vi "obwiednia_final.vi"() -> ()   [LabVIEW 2012]
uses:
  <vilib>/Analysis/3filter.llb/FIR Filter (DBL).vi
  <vilib>/Analysis/baseanly.llb/Mean (DBL).vi
  <vilib>/Utility/file.llb/Read From Spreadsheet File (DBL).vi
  <vilib>/addons/Sound and Vibration/Order Analysis/Fault Analysis/SVPO Envelope Detection (1 Ch DBL Array).vi
  <vilib>/Utility/file.llb/Write To Spreadsheet File (DBL).vi
  <vilib>/Analysis/4window.llb/Hamming Window (DBL).vi
  <vilib>/Analysis/NI_AALBase.lvlib
  <vilib>/Analysis/NI_AALPro.lvlib
  <vilib>/Analysis/NI_AAL_SigProc.lvlib
  <vilib>/addons/Sound and Vibration/Order Analysis/Fault Analysis/SoundVib_FaultAnalysis.lvlib
  <vilib>/gmath/NI_Gmath.lvlib
panel:
  out "Rozpoznano":bool
  out "Maks. indeks":i32
  out "Największy wsp.":dbl
  out "Współczynniki":dbl[](array[numeric])
  out "Odległość":dbl[](array[numeric])
  out "Waveform Graph 3":dbl[](graph)
  in  "Liczenie":bool
  in  "Pomiar":bool
  in  "stop":bool
  out "Signal energy":dbl
  out "Frames":dbl[][](array[numeric])
  out "Przekroczenie progu":bool
  out "Tablica ramek":dbl[](graph)
  out "number of columns":i32
  out "number of rows":i32
  out "Threshold Energy":dbl
  out "Diagram energii":dbl[](graph)
  out "size(s)":i32
  out "sum":dbl
  out "Length":dbl
  out "\"Wygładzona\" energia":dbl[](graph)
  out "max index":dbl
  out "min index":dbl
  out "Wypowiedź":dbl[](graph)
  out "Mowa":waveform(dbl)[](graph)
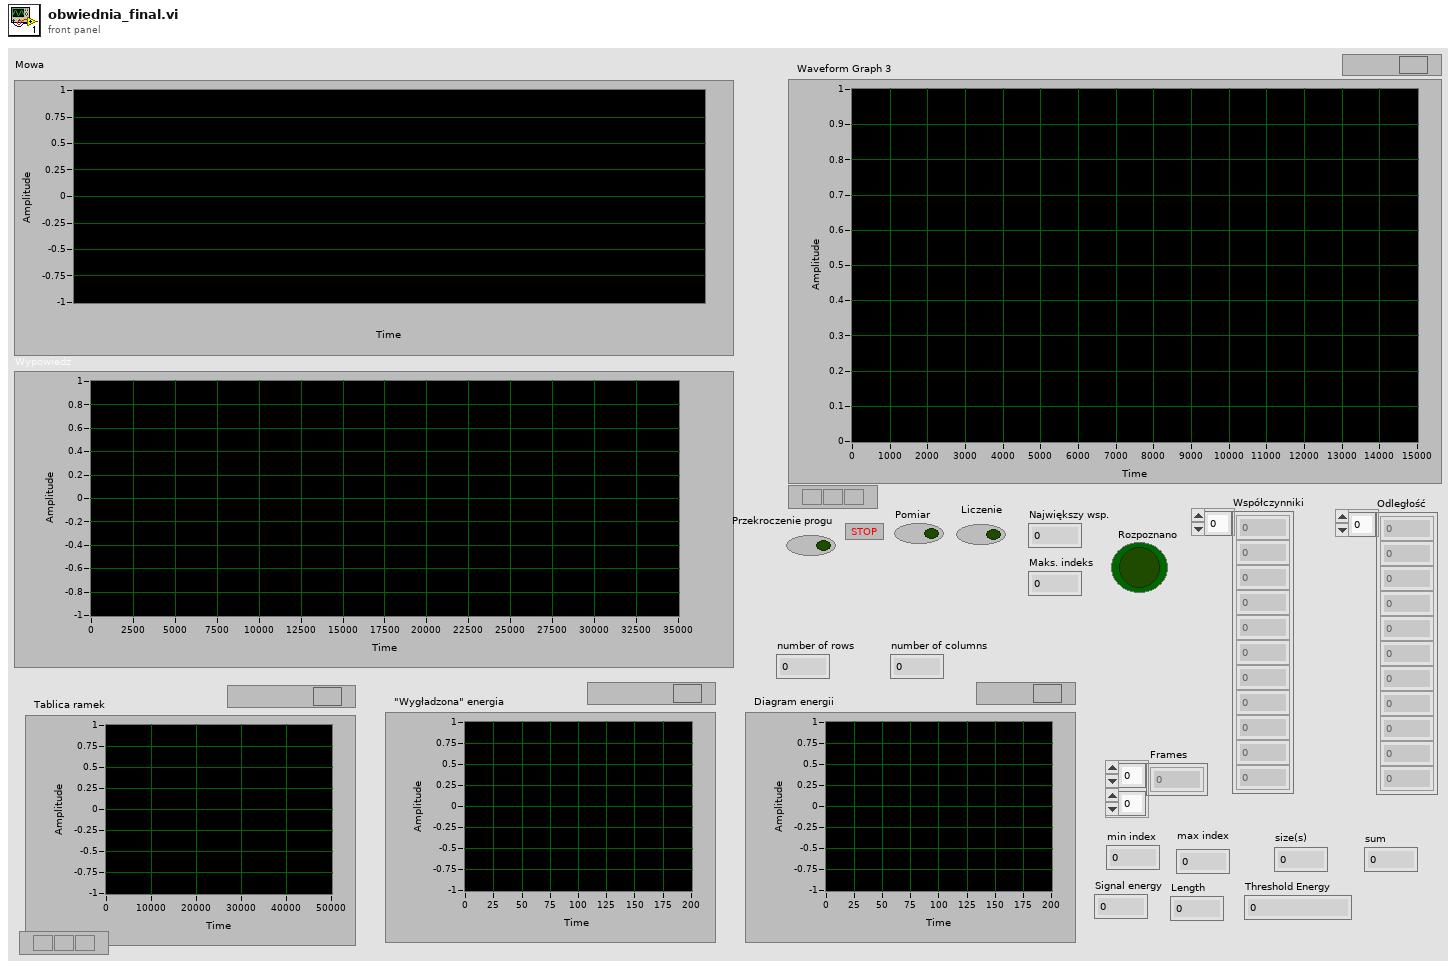
[diagram p1: front panel]
types:
  T1 = enum16{"open", "replace", "create", "open or create", "replace or create", "replace or create with confirmation"}
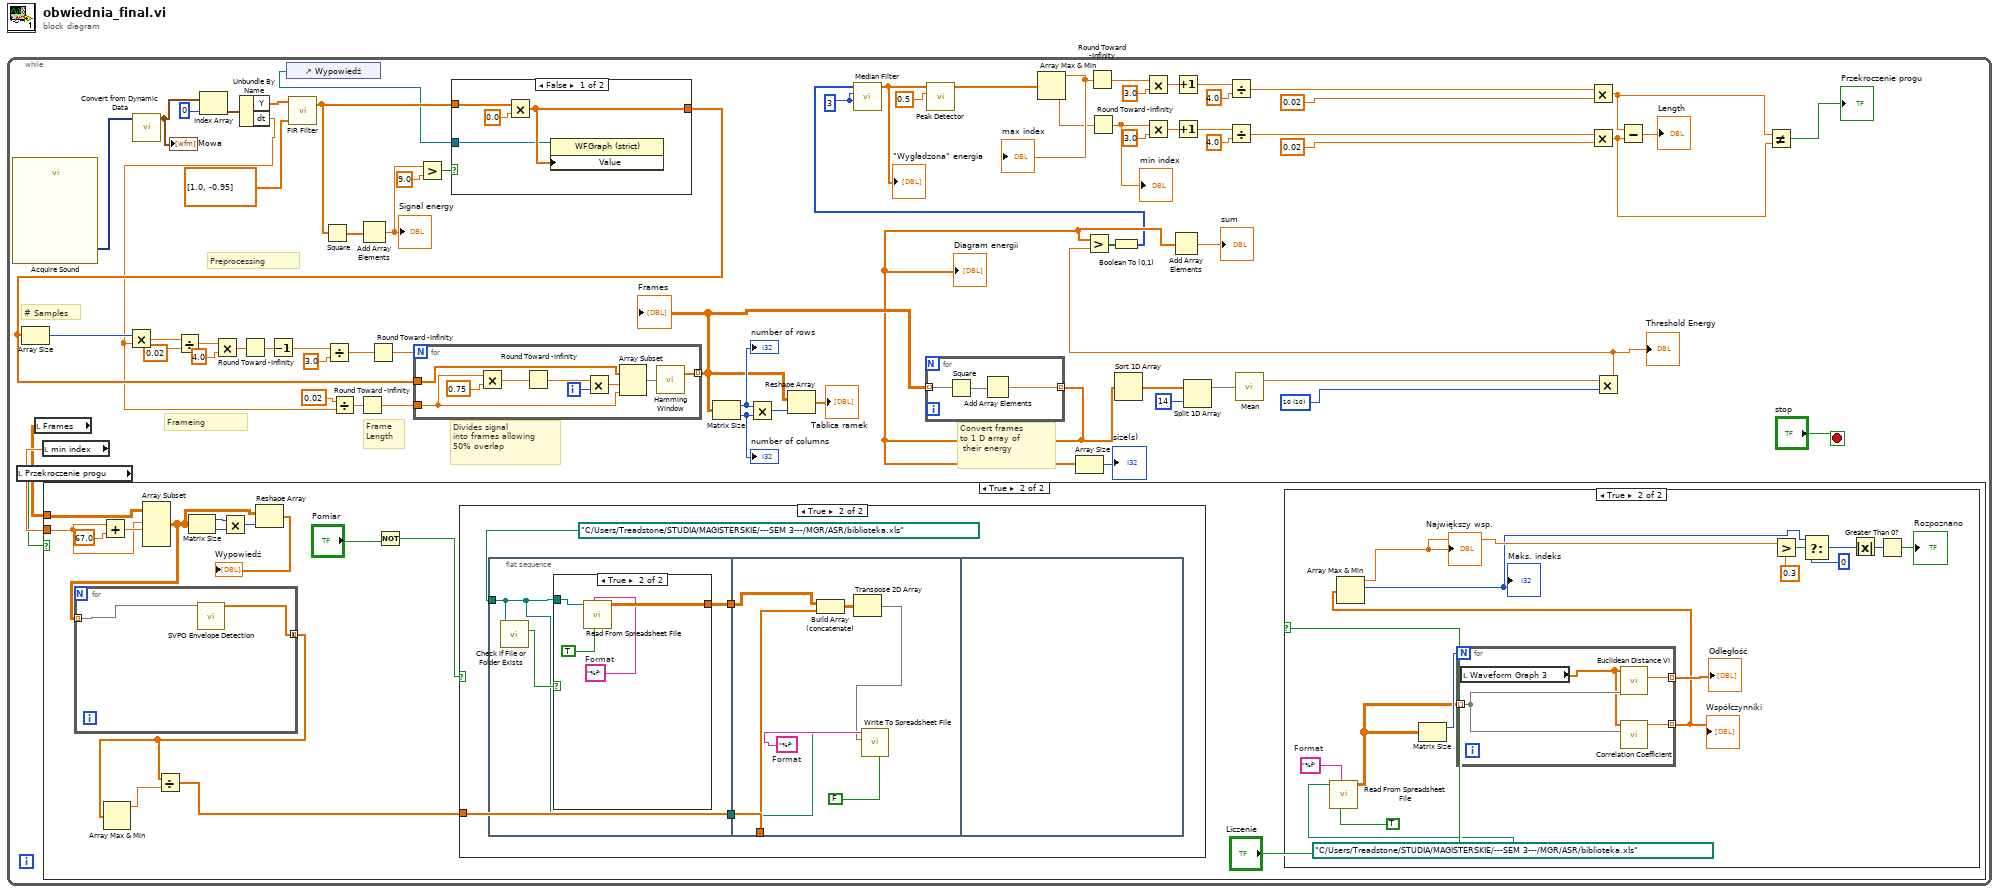
[diagram p0: block diagram]
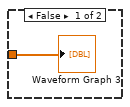
[diagram p3: hidden frame]
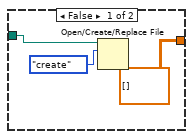
[diagram p4: hidden frame]
diagram:
  n1 = while {
    stop <- "stop" stop-if-true
    w16 = 3 ("right rank")
    w40 = u16 10 items=["5"=5, "6"=6, "7"=7, "9"=9, "10"=10]
    # "Frameing"
    # "Preprocessing"
    # "Convert frames \nto 1 D array of\n their energy"
    # "Divides signal \ninto frames allowing \n50% overlap"
    # "Frame \nLength"
    # "# Samples"
    n2 = call "Acquire Sound"() -> ("Data"=w72:dynamicdata)  [unwired: 18 in, 1 out]
    n3 = local read "Przekroczenie progu"() -> (w2:bool)
    n4 = local read "Frames"() -> (w3:dbl[][])
    n5 = local read "min index"() -> (w4:dbl)
    n6 = case shown="True" w2 {
      tunnel: w4 -> [_ w81]
      tunnel: w3 -> [_ w82]
      frame False {
      }
      frame True {
        n7 = Add(x=w81, y=67.0 ("x")) -> (x+y=w86:dbl)
        n8 = Array Subset(array=w82, index (row)=w81, length (row)=w86) -> (w79:dbl[][])  [unwired: 2 in]
        n9 = for {
          tunnel: w79 -> [w130] mode=indexing
          tunnel: [w129] -> w77 mode=concatenating
          n10 = call-poly <vilib>:"SVPO Envelope Detection.vi"("scaled signal [EU]"=w130) -> ("envelope signal [EU]"=w129:dbl[])  [unwired: 13 in, 1 out]
        }
        n11 = Array Max & Min(array=w77) -> (max value=w78:dbl)  [unwired: 3 out]
        n12 = Divide(x=w77, y=w78) -> (x/y=w75:dbl[])
        n13 = Matrix Size(0:w79) -> (1:w85:i32, 2:w84:i32)
        n14 = Multiply(x=w85, y=w84) -> (x*y=w83:i32)
        n15 = Reshape Array(w79, w83) -> (→"Wypowiedź":dbl[])
        n16 = Not(x="Pomiar") -> (.not. x?=w73:bool)
        n17 = case shown="True" w73 {
          tunnel: w75 -> [w88 w89]
          frame False {
            "Waveform Graph 3" <- w88
          }
          frame True {
            n18 = flat-sequence {
              tunnel: path "C:/Users/Treadstone/STUDIA/MAGISTERSKIE/---SEM 3---/MGR/ASR/biblioteka.xls" ("file path (dialog if empty)") -> [w93]
              tunnel: [w95] -> w92
              tunnel: [w93] -> w91
              tunnel: w92 -> [w103]
              tunnel: w89 -> [w106]
              tunnel: w91 -> [w107]
              frame #0 {
                n19 = call <vilib>:"Check if File or Folder Exists.vi"("path"=w93) -> ("file or folder exists?"=w94:bool)  [unwired: 8 in, 2 out]
                n20 = case shown="True" w94 {
                  tunnel: w93 -> [w98 w102]
                  tunnel: [dbl[][] [] ("all rows") w101] -> w95
                  frame False {
                    n21 = Open/Create/Replace File(file path (use dialog)=w98, operation (0:open)=T1."create") -> ()  [unwired: 4 in, 3 out]
                  }
                  frame True {
                    w100 = "%f"  # Format
                    n22 = call-poly <vilib>:"Read From Spreadsheet File.vi"("transpose (no:F)"=TRUE, "format (%.3f)"=w100, "file path (dialog if empty)"=w102) -> ("all rows"=w101:dbl[][])  [unwired: 4 in, 4 out]
                  }
                }
              }
              frame #1 {
                w109 = "%f"  # Format
                n23 = Build Array (concatenate)(w103, w106) -> (w105:dbl[][])
                n24 = Transpose 2D Array(2D array=w105) -> (transposed array=w104:dbl[][])
                n25 = call-poly <vilib>:"Write To Spreadsheet File.vi"("transpose? (no:F)"=FALSE, "format (%.3f)"=w109, "2D data"=w104, "file path (dialog if empty)"=w107) -> ()  [unwired: 4 in, 1 out]
              }
              frame #2 {
              }
            }
          }
        }
        n26 = case shown="True" "Liczenie" {
          frame False {
          }
          frame True {
            w123 = "%f"  # Format
            n27 = call-poly <vilib>:"Read From Spreadsheet File.vi"("transpose (no:F)"=TRUE, "format (%.3f)"=w123, "file path (dialog if empty)"=path "C:/Users/Treadstone/STUDIA/MAGISTERSKIE/---SEM 3---/MGR/ASR/biblioteka.xls") -> ("all rows"=w118:dbl[][])  [unwired: 4 in, 4 out]
            n28 = Matrix Size(0:w118) -> (1:w121:i32)  [unwired: 1 out]
            n29 = for {
              N: w121 -> [_]
              tunnel: w118 -> [w128] mode=indexing
              tunnel: [w126] -> w120 mode=indexing
              tunnel: [w125] -> w119 mode=indexing
              n30 = local read "Waveform Graph 3"() -> (w127:dbl[])
              n31 = call "Euclidean Distance VI.vi"("Reference"=w128, "Test"=w127) -> ("Dist"=w126:dbl)  [unwired: 9 in]
              n32 = call <vilib>:"Correlation Coefficient.vi"("Y"=w128, "X"=w127) -> ("correlation coefficient r"=w125:dbl)  [unwired: 8 in, 1 out]
            }
            "Odległość" <- w120
            "Współczynniki" <- w119
            n33 = Array Max & Min(array=w119) -> (max value=w111:dbl, max index (indices)=w110:i32)  [unwired: 2 out]
            "Największy wsp." <- w111
            "Maks. indeks" <- w110
            n34 = Greater?(x=w111, y=0.3) -> (0:w117:bool)
            n35 = Select(t=w110, s=w117, f=0) -> (s? t:f=w115:i32)
            n36 = Absolute Value(x=w115) -> (abs(x)=w114:i32)
            n37 = Greater Than 0?(x=w114) -> (x > 0?=→"Rozpoznano":bool)
          }
        }
      }
    }
    n38 = call "Convert from Dynamic Data"("Dynamic Data Type"=w72) -> ("Array of Waveform"=w1:waveform(dbl)[])  [unwired: 3 in]
    "Mowa" <- w1
    n39 = Index Array(array=w1, index=0) -> (element=w62:waveform(dbl))
    n40 = Unbundle By Name(w62) -> ("Y"=w61:dbl[], "dt"=w41:dbl)
    n41 = control-ref of="Wypowiedź"() -> (w5:refnum<vi>)
    n42 = call-poly <vilib>:"FIR Filter.vi"("FIR Coefficients"=dbl[] [1.0, -0.95], "X"=w61) -> ("Filtered X"=w70:dbl[])  [unwired: 2 in, 1 out]
    n43 = Square(x=w70) -> (x^2=w66:dbl[])
    n44 = Divide(x=0.02, y=w41) -> (x/y=w47:dbl)
    n45 = Round Toward -Infinity(1:w47) -> (0:w48:dbl)
    n46 = Add Array Elements(numeric array=w66) -> (sum=w68:dbl)
    "Signal energy" <- w68
    n47 = Greater?(x=w68, y=9.0) -> (0:w69:bool)
    n48 = case shown="False" w69 {
      tunnel: w70 -> [w145 w147]
      tunnel: [w144 w147] -> w42
      tunnel: w5 -> [w143 _]
      frame False {
        n49 = Multiply(x=w145, y=0.0) -> (x*y=w144:dbl[])
        n50 = property class="WFGraph (strict)"(reference=w143, "Value"=w144) -> ()  [unwired: 1 in, 2 out]
      }
      frame True {
      }
    }
    n51 = Array Size(array=w42) -> (size(s)=w60:i32)
    n52 = Multiply(x=w60, y=w41) -> (x*y=w58:dbl)
    n53 = Divide(x=w58, y=0.02) -> (x/y=w54:dbl)
    n54 = Multiply(x=w54, y=4.0) -> (x*y=w53:dbl)
    n55 = Round Toward -Infinity(1:w53) -> (0:w56:dbl)
    n56 = Decrement(x=w56) -> (x-1=w51:dbl)
    n57 = Divide(x=w51, y=3.0) -> (x/y=w50:dbl)
    n58 = Round Toward -Infinity(1:w50) -> (0:w49:dbl)
    n59 = for {
      N: w49 -> [_]
      tunnel: w42 -> [w142]
      tunnel: w48 -> [w139]
      tunnel: [w134] -> w32 mode=indexing
      i -> [w141]
      n60 = Multiply(x=w139, y=0.75 ("x")) -> (x*y=w137:dbl)
      n61 = Round Toward -Infinity(1:w137) -> (0:w136:dbl)
      n62 = Multiply(x=w136, y=w141) -> (x*y=w138:dbl)
      n63 = Array Subset(array=w142, index=w138, length=w139) -> (w135:dbl[])
      n64 = call-poly <vilib>:"Hamming Window.vi"("X"=w135) -> ("Windowed X"=w134:dbl[])  [unwired: 1 out]
    }
    "Frames" <- w32
    n65 = Matrix Size(0:w32) -> (1:w46:i32, 2:w45:i32)
    "number of columns" <- w45
    "number of rows" <- w46
    n66 = Multiply(x=w46, y=w45) -> (x*y=w44:i32)
    n67 = Reshape Array(w32, w44) -> (→"Tablica ramek":dbl[])
    n68 = for {
      tunnel: w32 -> [w133] mode=indexing
      tunnel: [w131] -> w9 mode=indexing
      n69 = Square(x=w133) -> (x^2=w132:dbl[])
      n70 = Add Array Elements(numeric array=w132) -> (sum=w131:dbl)
    }
    "Diagram energii" <- w9
    n71 = Array Size(array=w9) -> (size(s)=→"size(s)":i32)
    n72 = Sort 1D Array(array=w9) -> (sorted array=w36:dbl[])
    n73 = Add Array Elements(numeric array=w9) -> (sum=→"sum":dbl)
    n74 = Split 1D Array(array=w36, index=14) -> (first subarray=w34:dbl[])  [unwired: 1 out]
    n75 = call-poly <vilib>:"Mean.vi"("X"=w34) -> ("mean"=w33:dbl)  [unwired: 1 out]
    n76 = Multiply(x=w33, y=w40) -> (x*y=w39:dbl)
    "Threshold Energy" <- w39
    n77 = Greater?(x=w9, y=w39) -> (0:w38:bool[])
    n78 = Boolean To (0,1)(Boolean=w38) -> (0, 1=w6:i16[])
    n79 = call <vilib>:"Median Filter.vi"("right rank"=w16, "left rank"=w16, "X"=w6) -> ("Filtered X"=w13:dbl[])  [unwired: 7 in, 1 out]
    "\"Wygładzona\" energia" <- w13
    n80 = call <vilib>:"Peak Detector.vi"("threshold"=0.5, "X"=w13) -> ("Locations"=w15:dbl[])  [unwired: 5 in, 4 out]
    n81 = Array Max & Min(array=w15) -> (max value=w17:dbl, min value=w12:dbl)  [unwired: 2 out]
    "max index" <- w17
    n82 = Round Toward -Infinity(1:w17) -> (0:w30:dbl)
    n83 = Round Toward -Infinity(1:w12) -> (0:w11:dbl)
    "min index" <- w11
    n84 = Multiply(x=w30, y=3.0) -> (x*y=w19:dbl)
    n85 = Multiply(x=w11, y=3.0) -> (x*y=w28:dbl)
    n86 = Increment(x=w19) -> (x+1=w20:dbl)
    n87 = Increment(x=w28) -> (x+1=w27:dbl)
    n88 = Divide(x=w20, y=4.0) -> (x/y=w22:dbl)
    n89 = Divide(x=w27, y=4.0) -> (x/y=w25:dbl)
    n90 = Multiply(x=w22, y=0.02) -> (x*y=w8:dbl)
    n91 = Multiply(x=w25, y=0.02) -> (x*y=w7:dbl)
    n92 = Subtract(x=w8, y=w7) -> (x-y=→"Length":dbl)
    n93 = Not Equal?(x=w8, y=w7) -> (x != y?=→"Przekroczenie progu":bool)
  }
